vi "Send SystemInfo_UI.vi"(7 "Message Priority (Normal)":T2=enum."Normal", 8 "error in (no error)":errorcluster, 10 "SystemInit\ndata":T1, 11 "Message Enqueuer":refnum<class "Message Enqueuer.lvclass">) -> (0 "error out":errorcluster, 3 "Message Enqueuer out":refnum<class "Message Enqueuer.lvclass">)   [LabVIEW 2019, in "ZenGage v3.0 UI.lvlib" / "SystemInfo_UI.lvclass"]
doc: "This VI sends the message to an actor."
uses:
  SystemInfo_UI.lvclass
  <vilib>/ActorFramework/Message Enqueuer/Message Enqueuer.lvclass
  C:/Program Files/National Instruments/LabVIEW 2019/vi.lib/ActorFramework/Message/Message.lvclass
  <vilib>/ActorFramework/Message Enqueuer/Message Priority.ctl
  User Interface Actor/Type Definitions/JSON Read/Data initialization.ctl
  User Interface Actor/ZenGage v3.0 UI.lvclass
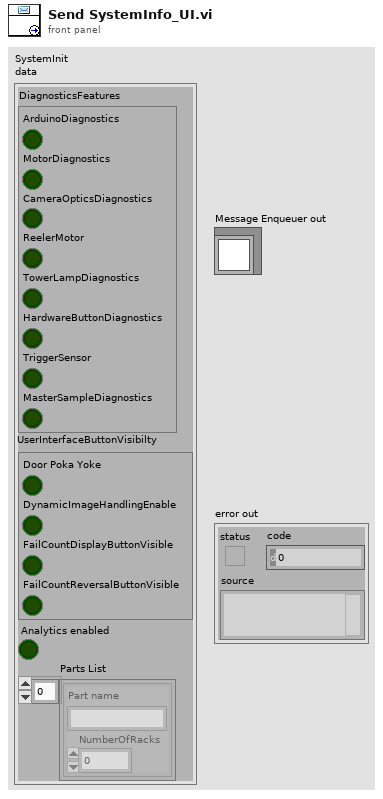
[diagram p1: front panel]
types:
  T1 = typedef "ZenGage v3.0 UI.lvclass/Data initialization.ctl" = cluster{"DiagnosticsFeatures":cluster{"ArduinoDiagnostics":bool, "MotorDiagnostics":bool, "CameraOpticsDiagnostics":bool, "ReelerMotor":bool, "TowerLampDiagnostics":bool, "HardwareButtonDiagnostics":bool, "TriggerSensor":bool, "MasterSampleDiagnostics":bool}, "UserInterfaceButtonVisibilty":cluster{"Door Poka Yoke":bool, "DynamicImageHandlingEnable":bool, "FailCountDisplayButtonVisible":bool, "FailCountReversalButtonVisible":bool}, "Analytics enabled":bool, "Parts List":cluster{"Part name":string, "NumberOfRacks":u8}[]}
  T2 = typedef "Actor Framework.lvlib/Message Enqueuer.lvclass/Message Priority.ctl" = enum16{"Low", "Normal", "High"}
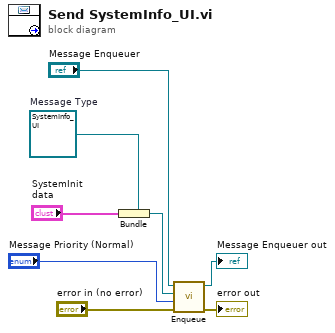
[diagram p0: block diagram]
diagram:
  w5 = refnum<class "SystemInfo_UI.lvclass"> refnum  # Message Type
  n1 = Bundle(cluster=w5, "SystemInit\ndata") -> (w4:refnum<class "SystemInfo_UI.lvclass">)
  n2 = call <vilib>:"Enqueue.vi"("error in (no error)"="error in (no error)", "Message Priority (Normal)"="Message Priority (Normal)", "Message"=w4, "Message Enqueuer in"="Message Enqueuer") -> ("error out"=→"error out":errorcluster, "Message Enqueuer out"=→"Message Enqueuer out":refnum<class "Message Enqueuer.lvclass">)  [unwired: 6 in]
